vi "Calcula flecha.vi"() -> ()   [LabVIEW 2020]
doc: "Cálculo da flecha para vão nivelado e desnivelado"
panel:
  in  "ps":dbl
  in  "T0s":dbl
  in  "As":dbl
  out "Fs":dbl
  out "Fc":dbl
  in  "Ac":dbl
  in  "T0c":dbl
  in  "pc":dbl
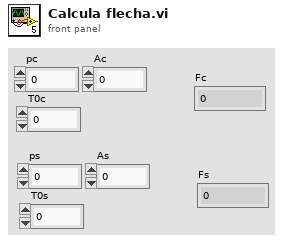
[diagram p1: front panel]
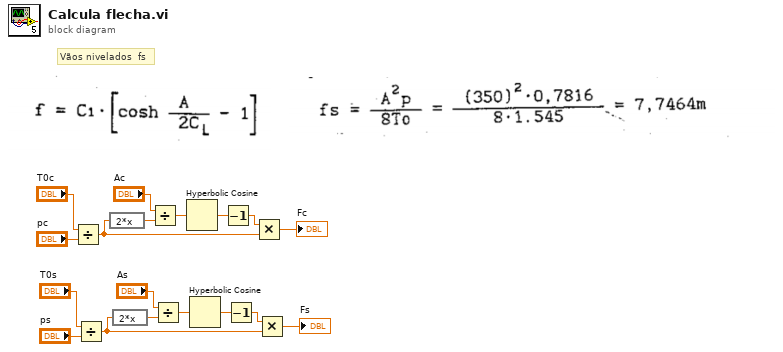
[diagram p0: block diagram]
diagram:
  # "Vãos nivelados  fs"
  n1 = Divide(x="T0c", y="pc") -> (x/y=w12:dbl)
  n2 = Divide(x="T0s", y="ps") -> (x/y=w7:dbl)
  n3 = expression code="2*x"(w12) -> (w13:dbl)
  n4 = expression code="2*x"(w7) -> (w6:dbl)
  n5 = Divide(x="Ac", y=w13) -> (x/y=w15:dbl)
  n6 = Divide(x="As", y=w6) -> (x/y=w4:dbl)
  n7 = Hyperbolic Cosine(1:w15) -> (0:w16:dbl)
  n8 = Hyperbolic Cosine(1:w4) -> (0:w3:dbl)
  n9 = Decrement(x=w16) -> (x-1=w11:dbl)
  n10 = Decrement(x=w3) -> (x-1=w8:dbl)
  n11 = Multiply(x=w11, y=w12) -> (x*y=→"Fc":dbl)
  n12 = Multiply(x=w8, y=w7) -> (x*y=→"Fs":dbl)
